vi "Check DB Connection.vi"(8 "Error In":errorcluster, 10 "Connection String":string="Provider=SQLOLEDB.1;Password=123456789;Persist Security Info=True;User ID=INO;Initial Catalog=OMS;Data Source=192.168.150.110,1433;Extended Properties=\"MultipleActiveResultSets=True\";Network Library=DBMSSOCN\n", 11 "UDL File":path=path "D:/TFS-Labview/NI 2019/Low Level Projects-2020-12-07/Low Level Projects/DB/LV_DB.udl" caption="UDL File (if blank, use Connection String)") -> (0 "Error Out":errorcluster, 3 "OK":bool)   [LabVIEW 2019]
doc: "Checks for a database connection at the UDL file you specify."
panel:
  in  "ADODB._Connection":refnum<k7>
  # "To create a UDL file, for the Database, please follow the steps below on TestStand:\n1. Go to Configure>>Results Processing.\n2. On the Database line, click on Advanced Settings (tool icon).\n3. Click Save .udl File and save it to your PC.\n4.  In this VI, load the .udl FIle you have just created into the control above \"UDL File\"."
  # "LED lights up if the connection is sucessful."
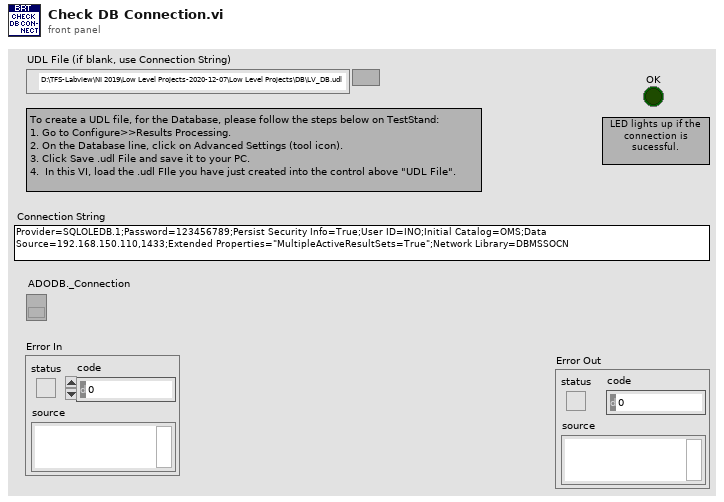
[diagram p1: front panel]
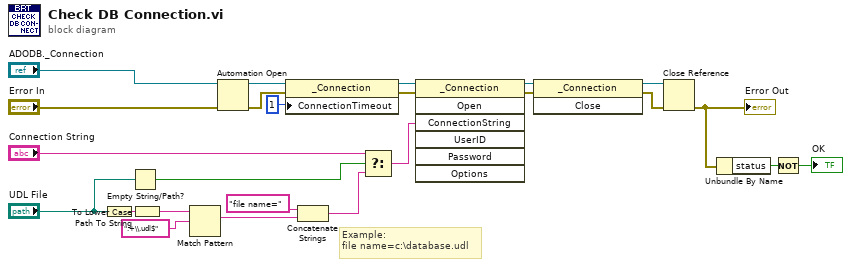
[diagram p0: block diagram]
diagram:
  # "Example:\nfile name=c:\\database.udl"
  n1 = Path To String(path="UDL File") -> (string=w13:string)
  n2 = Empty String/Path?(string/path="UDL File") -> (empty?=w7:bool)
  n3 = To Lower Case(string=w13) -> (all lower case string=w11:string)
  n4 = Match Pattern(string=w11, regular expression=".+\\.udl$") -> (match substring=w10:string)  [unwired: 4 out]
  n5 = Automation Open(error in (no error)="Error In", Automation Refnum="ADODB._Connection") -> (Automation Refnum=w17:refnum<k7>, error out=w16:errorcluster)  [unwired: 2 out]
  n6 = property class="_Connection"(reference=w17, error in=w16, "ConnectionTimeout"=1) -> (reference out=w19:refnum<k7>, error out=w20:errorcluster)
  n7 = Concatenate Strings("file name=" ("Substring"), w10) -> (w9:string)
  n8 = Select(t="Connection String", s=w7, f=w9) -> (s? t:f=w5:string)
  n9 = invoke class="_Connection" method="Open"(reference=w19, error in=w20, "ConnectionString"=w5) -> (reference out=w22:refnum<k7>, error out=w21:errorcluster)  [unwired: 4 in, 5 out]
  n10 = invoke class="_Connection" method="Close"(reference=w22, error in=w21) -> (reference out=w23:refnum<k7>, error out=w24:errorcluster)  [unwired: 1 in, 1 out]
  n11 = Close Reference(reference=w23, error in (no error)=w24) -> (error out=w3:errorcluster)
  "Error Out" <- w3
  n12 = Unbundle By Name(w3) -> ("status"=w2:bool)
  n13 = Not(x=w2) -> (.not. x?=→"OK":bool)
